vi "AzCamGlobals.vi"() -> ()   [LabVIEW 2014]
panel:
  in  "Tab Control":enum32{"Flags", "Admin", "Files"}(tab)=enum."Admin"
  out "ShowClientCommands":bool=TRUE
  out "DisplayImage":bool=TRUE
  out "ReadTemps":bool
  out "TelescopeEnabled":bool
  out "InstrumentEnabled":bool
  out "CloseAzCamServer":bool
  out "PanelLock":bool
  out "ShutDown":bool
  out "SocketOpen":bool
  out "TestImage":bool=TRUE
  out "UserWarnings":bool
  out "ClearArray":bool=TRUE
  out "UseSound":bool=TRUE
  out "Prompt4Title":bool
  out "StartupReset":bool
  out "TotalPixels":i32
  out "ExposureSequenceFlush":i32
  out "ExposureSequenceDelay":dbl format="%_3g"
  out "ExposureSequenceTotal":i32
  out "AzCamErrorCode":i32
  in  "AzCamImageWriterPort":i32=2406
  in  "InstrumentVI":string
  in  "ClientHostName":string="quantum.itl.arizona.edu"
  in  "LastTitle":string
  in  "Version":string="12Feb13"
  in  "ImageFormat":T1(ring)=enum."Extended FITS"
  in  "ServerPort":i32=2402
  in  "ServerName":string="localhost"
  in  "ConnectionID":refnum<k5>
  in  "AzCamToolRef":refnum<vi>
  out "OS":i32=3
  in  "ImageTypes":string[](array[string])=["zero", "object", "flat", "dark", "ramp"]
  in  "ImageType":string="zero"
  out "ImageHeaderFile":path
  out "ClientConfigFile":path
  in  "AzCamImageWriterPath":path=path "C:/AzCam/Plugins/AzCamImageWriter/AzCamImageWriter.py"
  in  "AzCamConsolePath":path=path "C:/AzCam/Plugins/AzCamLog/AzCamLog.py"
  in  "RootDir":path=path "C:/AzCam/Plugins/AzCamTool"
  in  "Filename":string="c:/data/test.fits"
  in  "SoundReadout":path=path "C:/AzCam/Plugins/AzCamTool/Sounds/snd_readout_finished.wav"
  in  "SystemFolder":path=path "C:/azcam/systems/soguiders"
  out "AzCamToolParFile":path=path "C:/AzCam/Plugins/AzCamTool/AzCamToolPars.ini"
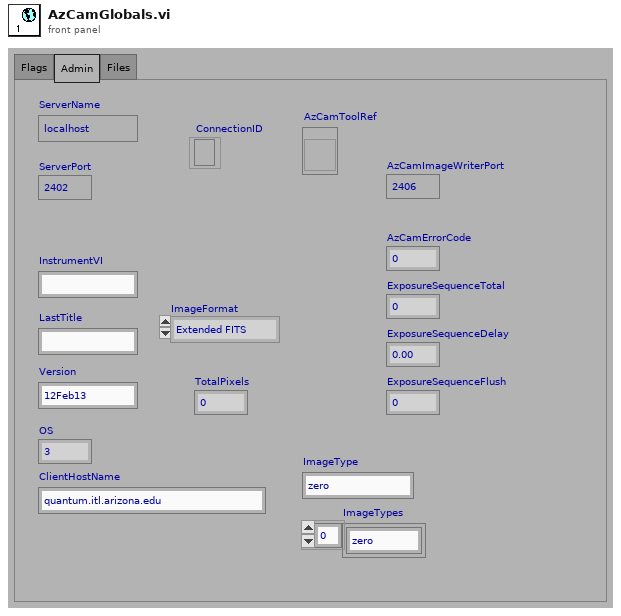
[diagram p1: front panel]
types:
  T1 = enum16{"FITS", "Extended FITS", "Binary", "TIFF", "JPEG", "GIF", "Thumbnail"}
diagram:
